vi "Triangular Probability Density Noise.vi"(10 "amplitude":dbl=1.0 format="%0.2f", 11 "samples":i32=128) -> (3 "TPDF noise":dbl[](array[numeric]))   [LabVIEW 2022 SP3]
uses:
  <vilib>/Analysis/NI_AALBase.lvlib
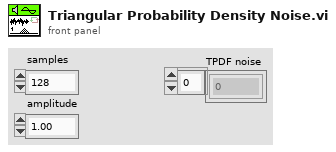
[diagram p1: front panel]
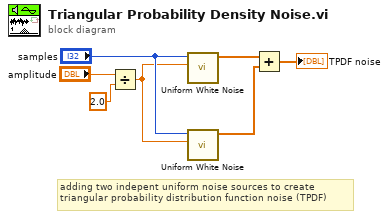
[diagram p0: block diagram]
diagram:
  # "adding two indepent uniform noise sources to create\ntriangular probability distribution function noise (TPDF)"
  n1 = Divide(x="amplitude", y=2.0) -> (x/y=w4:dbl)
  n2 = call <vilib>:"Uniform White Noise.vi"("amplitude"=w4, "samples"="samples") -> ("uniform white noise"=w3:dbl[])  [unwired: 8 in, 1 out]
  n3 = call <vilib>:"Uniform White Noise.vi"("amplitude"=w4, "samples"="samples") -> ("uniform white noise"=w2:dbl[])  [unwired: 8 in, 1 out]
  n4 = Add(x=w3, y=w2) -> (x+y=→"TPDF noise":dbl[])
